vi "Particle_Setting_UI.vi"(4 "ForCalCalculaton In":T1, 6 "Analysis_Setting IN":T2 {"Analysis_Type" items=["None", "PatternMatch", "Edge Detection", "Barcode 1D", "Barcode 2D", "Clamp", "Clamp MAX", "Particle", "Histogram", "Straight Edge", "Circle", "Shape Detect", "OCR", "Contour", "ColorMatch"]}, 8 "error in (no error)":errorcluster, 9 "ProjectName":string, 10 "ROI List IN":refnum<vi>, 11 "Vision_Image":T1(plugin-control)) -> (0 "error out":errorcluster, 1 "Cancel?":bool, 2 "TempAnalysisResult":variant, 3 "Analysis_Setting":T2 {"Analysis_Type" items=["None", "PatternMatch", "Edge Detection", "Barcode 1D", "Barcode 2D", "Clamp", "Clamp MAX", "Particle", "Histogram", "Straight Edge", "Circle", "Shape Detect", "OCR", "Contour", "ColorMatch"]})   [LabVIEW 2015]
uses:
  Controls/Analysis_Setting.ctl
  Controls/Analysis_Type.ctl
  <vilib>/vision/Image Controls.llb/IMAQ Image.ctl
  Controls/_UI Command Cluster/Particle_UI Command Cluster.ctl
  Controls/Particle/Analysis_Particle_Parameter.ctl
  <vilib>/vision/NI_Vision_Development_Module.lvlib
panel:
  in  "Selected Particle":i32=2 min=-1 max=34
  in  "Simulation":bool
  out "Numeric":i32
  in  "Done":bool
  in  "Particle_UI Command":T4(ring)
  in  "Cancel":bool
  in  "ParticleTab":T5(tab)
  in  "MaxParticle":i32=1
  in  "Connectivity 4/8 (8)":bool=TRUE
  out "Selected Particle Report":T6(array[cluster]) {"Orientation" format="%.2f"; "Center of Mass"."Y" format="%.2f"; "Center of Mass"."X" format="%.2f"}
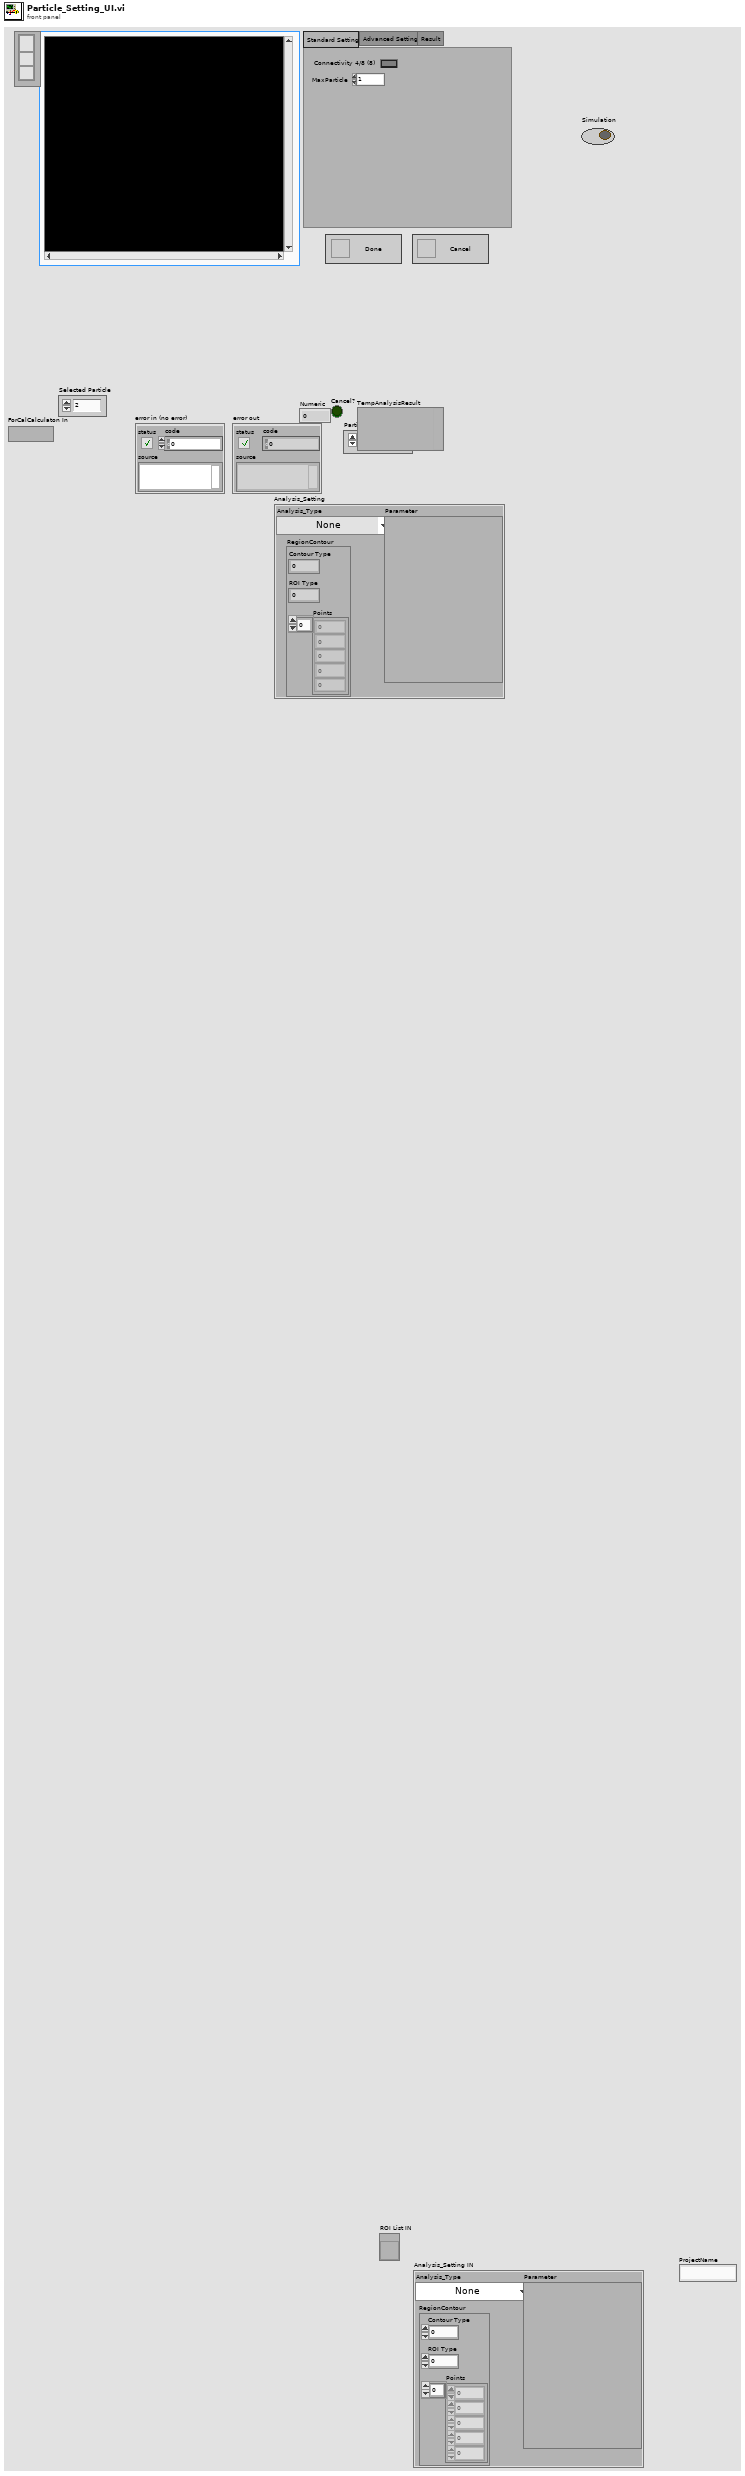
[diagram p1: front panel]
types:
  T1 = typedef "IMAQ Image.ctl" = refnum<image>
  T2 = typedef "Analysis_Setting.ctl" = cluster{"Analysis_Type":T3, "RegionContour":cluster{"Contour Type":u32, "ROI Type":u32, "Points":i32[]}, "Parameter":variant}
  T3 = typedef "Analysis_Type.ctl" = u16
  T4 = enum16{"Initialize", "Done", "Run Algorithm", "Cancel"}
  T5 = enum32{"Standard Setting", "Advanced Setting", "Result"}
  T6 = cluster{"Area":dbl, "Number of Holes":dbl, "Bounding Rect":cluster{"Left":dbl, "Top":dbl, "Right":dbl, "Bottom":dbl}, "Center of Mass":cluster{"X":dbl, "Y":dbl}, "Orientation":dbl, "Dimensions":cluster{"Width":dbl, "Height":dbl}}[]
  T7 = typedef "Particle_UI Command Cluster.ctl" = cluster{"Particle_UI Command":enum16{"Initialize", "Done", "Run Algorithm", "Cancel"}, "Selected Particle":i32, "Snap Simulation Mouse Down":bool, "Connectivity 4/8 (8)":bool, "MaxParticle":i32}
  T8 = typedef "IMAQ Line" = cluster{"Start X":i32, "Start Y":i32, "End X":i32, "End Y":i32}
  T9 = cluster{"Contour Type":u32, "ROI Type":u32, "Points":i32[]}
  T10 = typedef "Image Type" = u32
  T11 = typedef "Analysis_Particle_Parameter.ctl" = cluster{"Selected Particle":i32, "Connectivity 4/8 (8)":bool, "MaxParticle":i32}
  T12 = typedef "ROI Descriptor" = cluster{"Global Rectangle":i32[], "Contours":cluster{"ID":enum32{"External", "Internal"}, "Type":u32, "Coordinates":i32[]}[]}
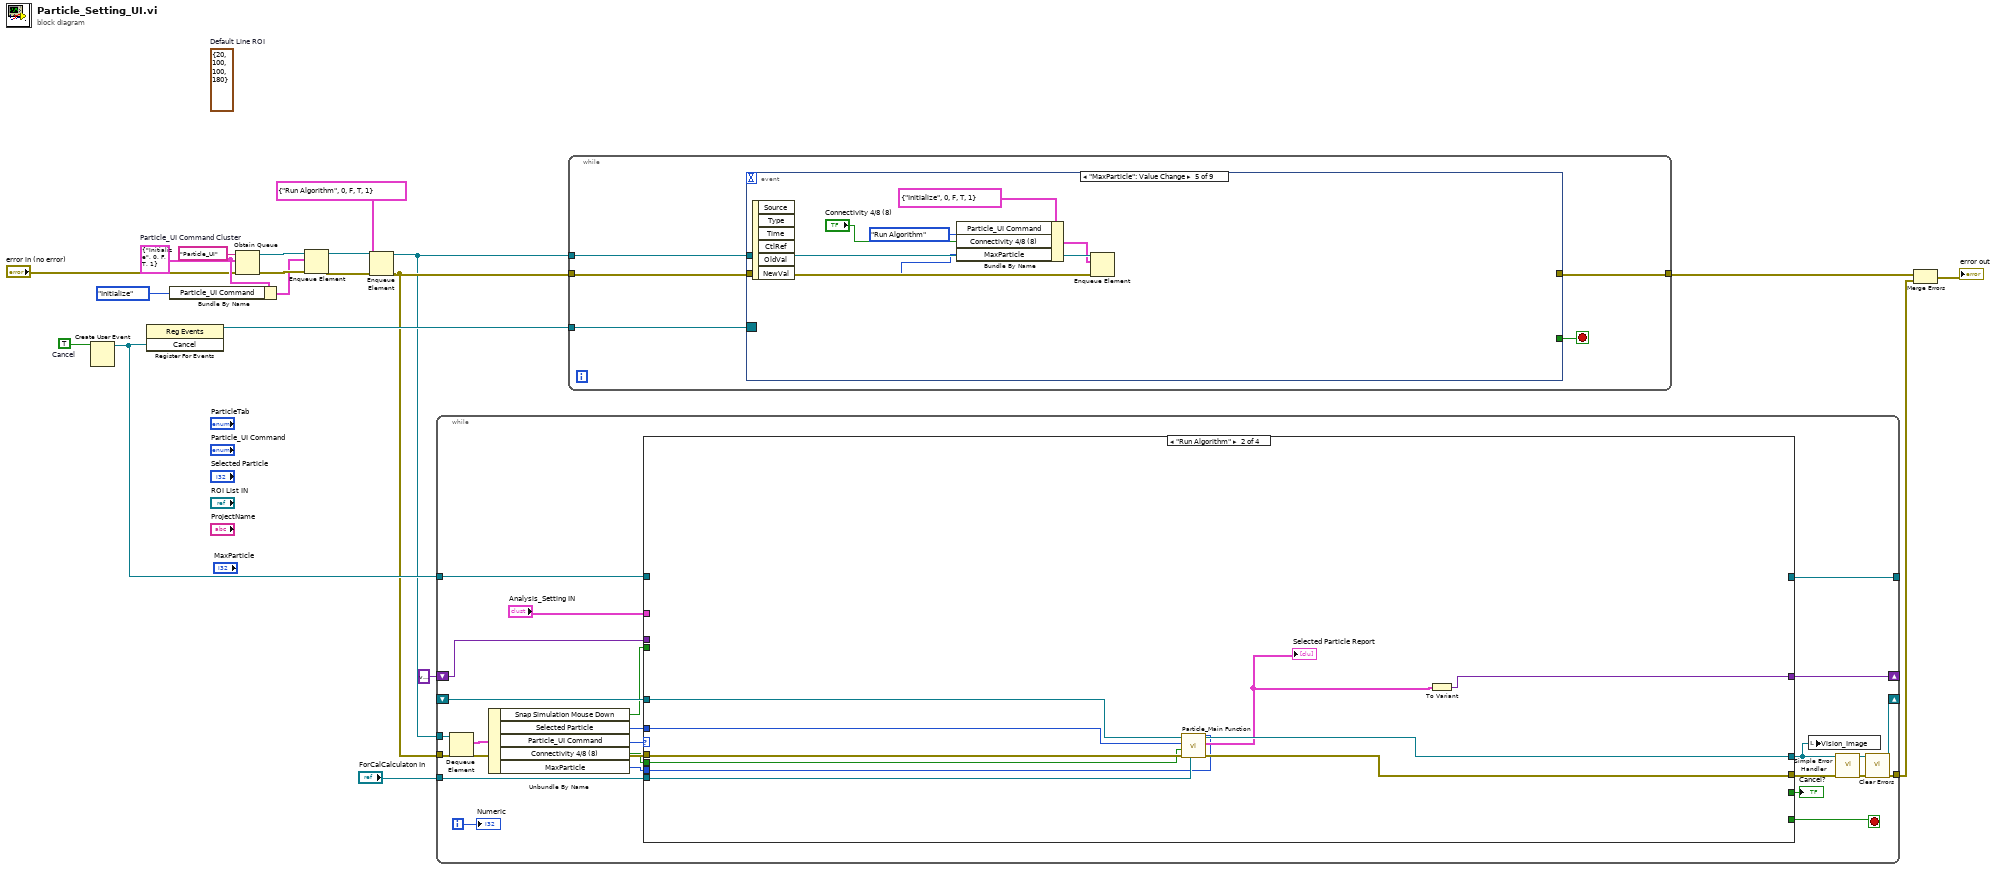
[diagram p0: block diagram]
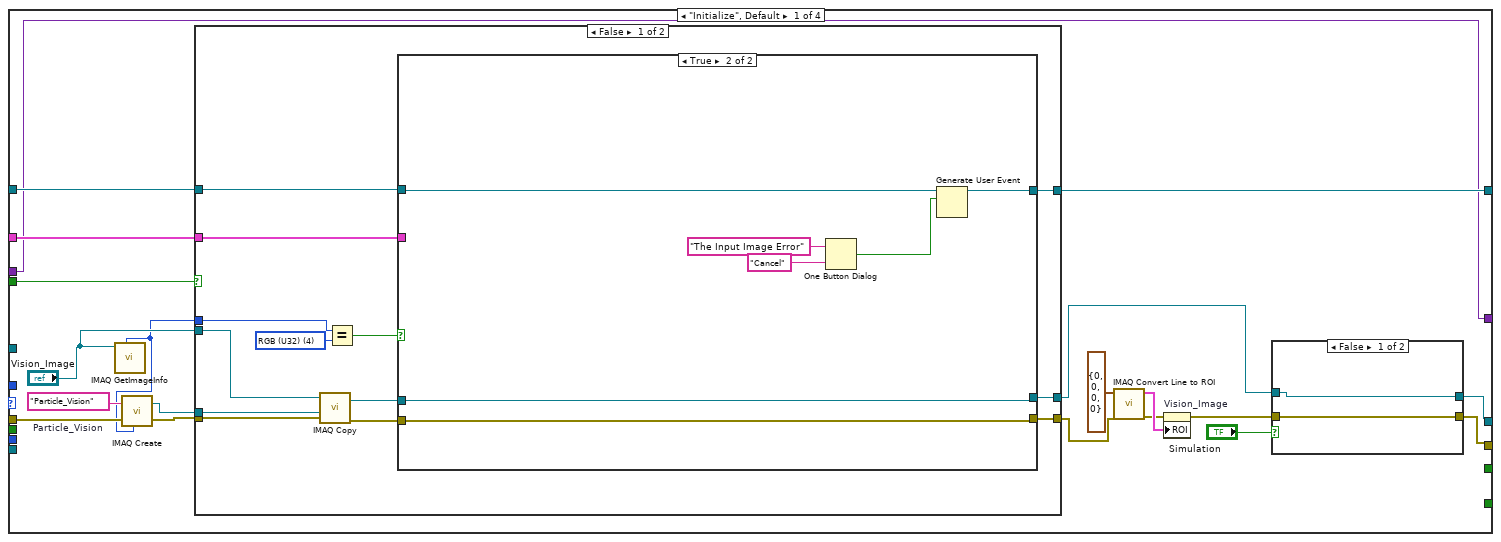
[diagram p2: hidden frame]
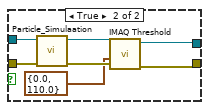
[diagram p3: hidden frame]
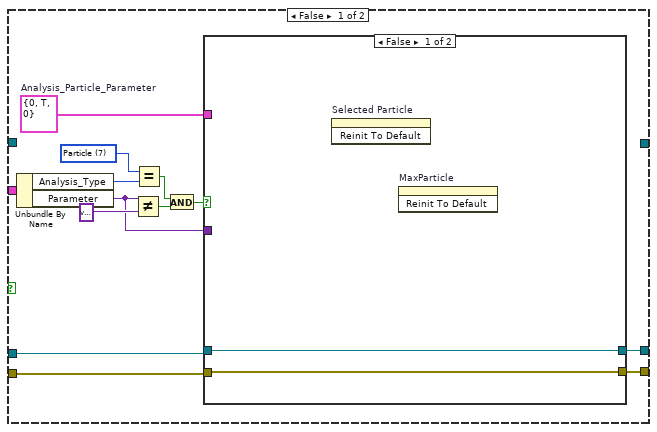
[diagram p4: hidden frame]
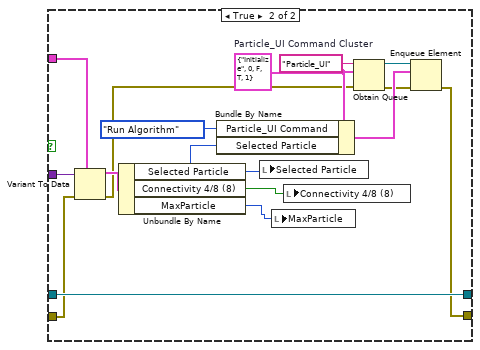
[diagram p5: hidden frame]
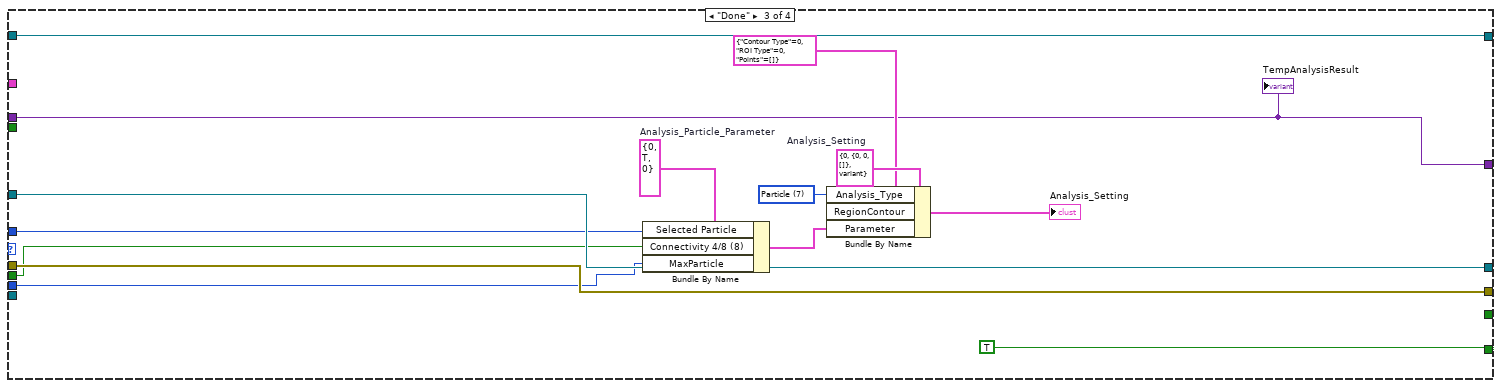
[diagram p7: hidden frame]
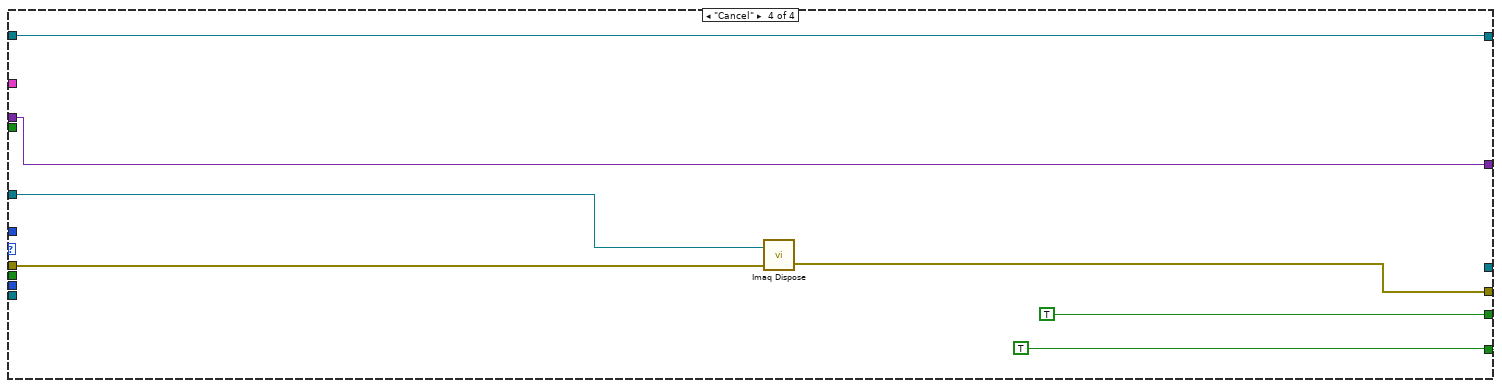
[diagram p8: hidden frame]
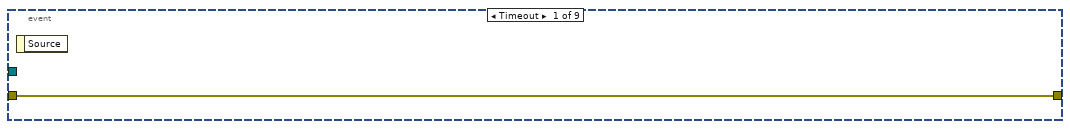
[diagram p9: hidden frame]
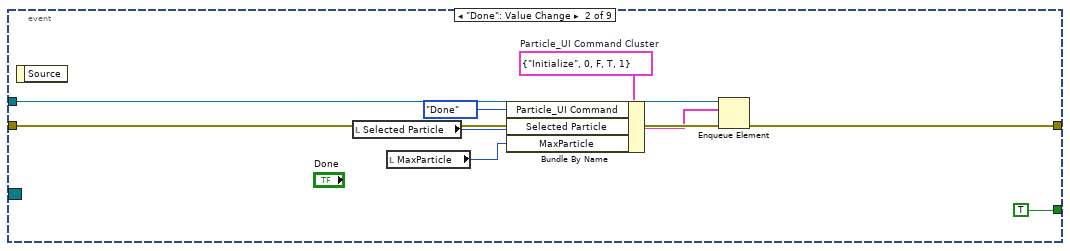
[diagram p10: hidden frame]
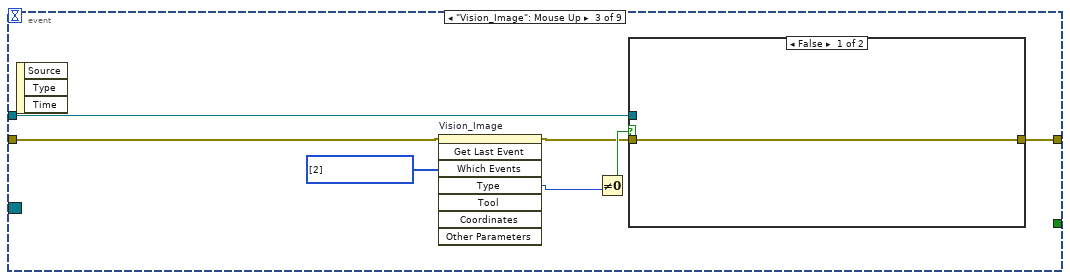
[diagram p11: hidden frame]
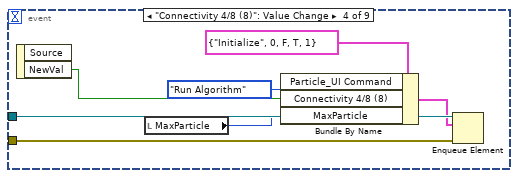
[diagram p13: hidden frame]
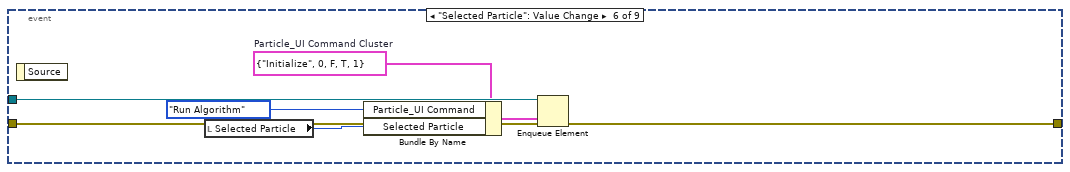
[diagram p14: hidden frame]
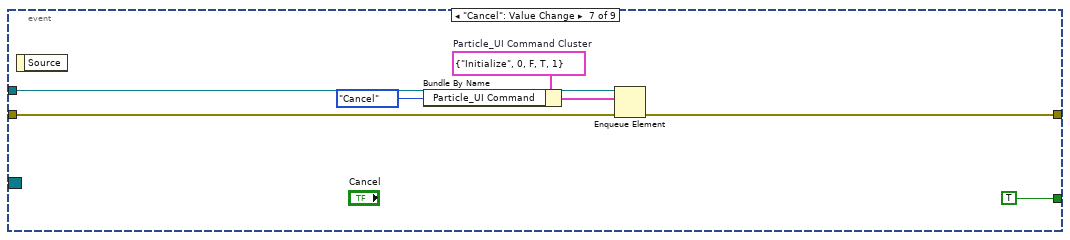
[diagram p15: hidden frame]
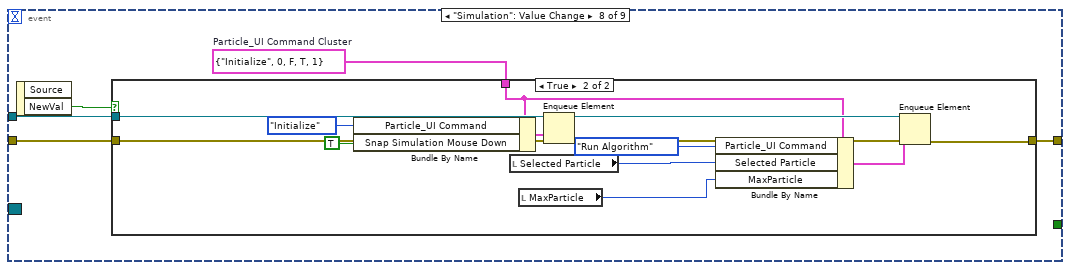
[diagram p16: hidden frame]
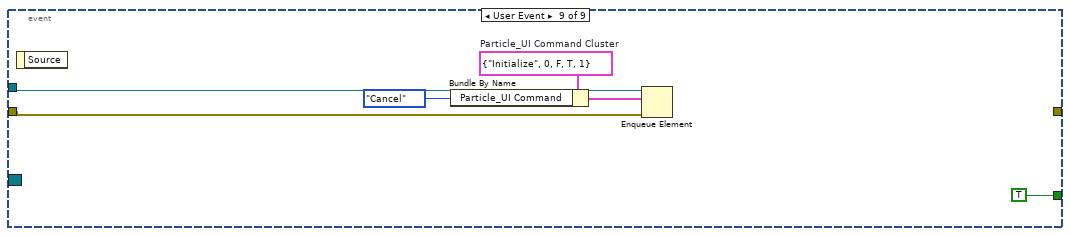
[diagram p18: hidden frame]
diagram:
  w10 = TRUE  # Cancel
  w13 = T7 {"Particle_UI Command"=enum."Initialize", "Selected Particle"=0, "Snap Simulation Mouse Down"=FALSE, "Connectivity 4/8 (8)"=TRUE, "MaxParticle"=1}  # Particle_UI Command Cluster
  (unwired) T8 {"Start X"=20, "Start Y"=100, "End X"=100, "End Y"=180}  # Default Line ROI
  n1 = Create User Event(user event datatype=w10) -> (user event=w8:refnum<user-event>)  [unwired: 1 in, 1 out]
  n2 = register-events(w8) -> (reference out=w9:refnum<event-registration>)  [unwired: 2 in, 1 out]
  n3 = Bundle By Name(cluster=w13, "Particle_UI Command"=T4."Initialize" ("Barcode 1D_UI Command")) -> (w14:T7)
  n4 = Obtain Queue(name (unnamed)="Particle_UI", element data type=w13, error in (no error)="error in (no error)") -> (queue out=w20:refnum<queue>, error out=w19:errorcluster)  [unwired: 2 in, 1 out]
  n5 = Enqueue Element(queue=w20, element=w14, error in (no error)=w19) -> (queue out=w5:refnum<queue>, error out=w7:errorcluster)  [unwired: 1 in, 1 out]
  n6 = Enqueue Element(queue=w5, element=T7 {"Particle_UI Command"=enum."Run Algorithm", "Selected Particle"=0, "Snap Simulation Mouse Down"=FALSE, "Connectivity 4/8 (8)"=TRUE, "MaxParticle"=1}, error in (no error)=w7) -> (queue out=w4:refnum<queue>, error out=w6:errorcluster)  [unwired: 1 in, 1 out]
  n7 = while {
    tunnel: w4 -> [w43]
    tunnel: w6 -> [w42]
    shift-right: [w35] -> _
    shift-left: _ -> [w37]
    tunnel: [w21] -> w16
    tunnel: w8 -> [w28]
    tunnel: [w27] -> _
    shift-right: [w26] -> _
    shift-left: variant ("Variant") -> [w25]
    tunnel: "ForCalCalculaton In" -> [w23]
    i -> [w36]
    stop <- w38 stop-if-true
    n8 = Dequeue Element(queue=w43, error in (no error)=w42) -> (element=w39:T7, error out=w40:errorcluster)  [unwired: 1 in, 2 out]
    n9 = Unbundle By Name(w39) -> ("Snap Simulation Mouse Down"=w31:bool, "Selected Particle"=w33:i32, "Particle_UI Command"=w41:T4, "Connectivity 4/8 (8)"=w24:bool, "MaxParticle"=w22:i32)
    n10 = case shown="\"Run Algorithm\"" w41 {
      tunnel: w40 -> [w62 w135 w147 w154]
      tunnel: [w49 w131 w147 w153] -> w30
      tunnel: [_ _ TRUE TRUE] -> w38
      tunnel: [w50 w132 w148 _] -> w35
      tunnel: w37 -> [_ w133 w148 w155]
      tunnel: [_ _ _ TRUE] -> w34
      tunnel: w33 -> [_ w134 w141 _]
      tunnel: "Analysis_Setting IN" -> [w61 _ _ _]
      tunnel: w31 -> [w53 _ _ _]
      tunnel: w28 -> [w48 _ w139 w151]
      tunnel: [w47 _ w139 w151] -> w27
      tunnel: [w44 w129 w138 w150] -> w26
      tunnel: w25 -> [w44 _ w138 w150]
      tunnel: w24 -> [_ w128 w137 _]
      tunnel: w23 -> [_ w127 _ _]
      tunnel: w22 -> [_ w126 w136 _]
      frame "Initialize", Default {
        w63 = "Particle_Vision"  # Particle_Vision
        n11 = call "IMAQ GetImageInfo"("Image"="Vision_Image") -> ("Image Type"=w45:T10)  [unwired: 3 in, 7 out]
        n12 = call "IMAQ Create"("Image Name"=w63, "Image Type"=w45, "error in (no error)"=w62) -> ("New Image"=w51:T1, "error out"=w52:errorcluster)  [unwired: 2 in]
        n13 = case shown="False" w53 {
          tunnel: w61 -> [w85 _]
          tunnel: [w84 w125] -> w54
          tunnel: [w83 w124] -> w55
          tunnel: w52 -> [w82 w124]
          tunnel: w51 -> [w81 w125]
          tunnel: w48 -> [w76 _]
          tunnel: [w75 _] -> w47
          tunnel: "Vision_Image" -> [w74 _]
          tunnel: w45 -> [w73 _]
          frame False {
            w78 = T10 4 items=["Grayscale (U8)", "Grayscale (I16)", "Grayscale (SGL)", "Complex (CSG)", "RGB (U32)", "HSL (U32)", "RGB (U64)", "Grayscale (U16)"] ("y")
            n14 = call "IMAQ Copy"("error in (no error)"=w82, "Image Dst"=w81, "Image Src"=w74) -> ("error out"=w80:errorcluster, "Image Dst Out"=w79:T1)  [unwired: 3 in]
            n15 = Equal?(x=w73, y=w78) -> (x = y?=w77:bool)
            n16 = case shown="True" w77 {
              tunnel: w85 -> [w91 _]
              tunnel: [w89 w117] -> w84
              tunnel: [w88 w118] -> w83
              tunnel: w80 -> [w87 w118]
              tunnel: w79 -> [w86 w117]
              tunnel: w76 -> [_ w120]
              tunnel: [_ w119] -> w75
              frame False {
                w90 = T11 {"Selected Particle"=0, "Connectivity 4/8 (8)"=TRUE, "MaxParticle"=0}  # Analysis_Particle_Parameter
                w96 = T3 7 items=["None", "PatternMatch", "Edge Detection", "Barcode 1D", "Barcode 2D", "Clamp", "Clamp MAX", "Particle", "Histogram", "Straight Edge", "Circle", "Shape Detect", "OCR", "Contour", "ColorMatch"] ("x")
                n17 = Unbundle By Name(w91) -> ("Analysis_Type"=w95:T3, "Parameter"=w92:variant)
                n18 = Not Equal?(x=w92, y=variant) -> (x != y?=w97:bool)
                n19 = Equal?(x=w96, y=w95) -> (x = y?=w98:bool)
                n20 = And(x=w98, y=w97) -> (x .and. y?=w93:bool)
                n21 = case shown="False" w93 {
                  tunnel: w87 -> [w99 w105]
                  tunnel: w86 -> [w100 w106]
                  tunnel: [w100 w106] -> w89
                  tunnel: [w99 w103] -> w88
                  tunnel: w92 -> [_ w116]
                  tunnel: w90 -> [_ w114]
                  frame False {
                    n22 = invoke on="Selected Particle" class="DigNum (strict)" method="Reinit To Default"() -> ()  [unwired: 3 in, 3 out]
                    n23 = invoke on="MaxParticle" class="DigNum (strict)" method="Reinit To Default"() -> ()  [unwired: 3 in, 3 out]
                  }
                  frame True {
                    w113 = T7 {"Particle_UI Command"=enum."Initialize", "Selected Particle"=0, "Snap Simulation Mouse Down"=FALSE, "Connectivity 4/8 (8)"=TRUE, "MaxParticle"=1}  # Particle_UI Command Cluster
                    n24 = Variant To Data(error in=w105, type=w114, Variant=w116) -> (data=w115:T11, error out=w104:errorcluster)
                    n25 = Unbundle By Name(w115) -> ("Selected Particle"=w107:i32, "Connectivity 4/8 (8)"=w102:bool, "MaxParticle"=w101:i32)
                    n26 = Bundle By Name(cluster=w113, "Particle_UI Command"=T4."Run Algorithm" ("Barcode 1D_UI Command"), "Selected Particle"=w107) -> (w112:T7)
                    n27 = local write "Selected Particle"(w107) -> ()
                    n28 = local write "MaxParticle"(w101) -> ()
                    n29 = local write "Connectivity 4/8 (8)"(w102) -> ()
                    n30 = Obtain Queue(name (unnamed)="Particle_UI", element data type=w113, error in (no error)=w104) -> (queue out=w108:refnum<queue>, error out=w109:errorcluster)  [unwired: 2 in, 1 out]
                    n31 = Enqueue Element(queue=w108, element=w112, error in (no error)=w109) -> (error out=w103:errorcluster)  [unwired: 1 in, 2 out]
                  }
                }
              }
              frame True {
                n32 = One Button Dialog(message="The Input Image Error", button name ("OK")="Cancel") -> (true=w121:bool)
                n33 = Generate User Event(user event=w120, event data cluster=w121) -> (user event out=w119:refnum<user-event>)  [unwired: 2 in, 1 out]
              }
            }
          }
          frame True {
          }
        }
        n34 = call "IMAQ Convert Line to ROI"("error in (no error)"=w55, "Line"=T8 {"Start X"=0, "Start Y"=0, "End X"=0, "End Y"=0}) -> ("error out"=w56:errorcluster, "ROI Descriptor"=w57:T12)  [unwired: 7 in]
        n35 = property on="Vision_Image" class="ImageControl"(error in=w56, "ROI"=w57) -> (error out=w59:errorcluster)  [unwired: 1 in, 1 out]
        n36 = case shown="False" "Simulation" {
          tunnel: [w65 w67] -> w49
          tunnel: [w64 w68] -> w50
          tunnel: w59 -> [w65 w72]
          tunnel: w54 -> [w64 w71]
          frame False {
          }
          frame True {
            n37 = call "Particle_Simulaation.vi"("error in (no error)"=w72, "Refnum in"=w71) -> ("error out"=w69:errorcluster, "Refnum out"=w70:T1)  [unwired: 8 in]
            n38 = call "IMAQ Threshold"("error in (no error)"=w69, "Range"=cluster{"Lower value":sgl, "Upper value":sgl} {"Lower value"=0.0, "Upper value"=110.0}, "Image Src"=w70) -> ("error out"=w67:errorcluster, "Image Dst Out"=w68:T1)  [unwired: 7 in]
          }
        }
      }
      frame "Run Algorithm" {
        n39 = call "Particle_Main Function.vi"("ForCalCalculaton In"=w127, "MAXParticle"=w126, "error in (no error)"=w135, "Connectivity 4/8 (8)"=w128, "Selected Particle"=w134, "Refnum in"=w133) -> ("error out"=w131:errorcluster, "Particle Report"=w130:T6, "Refnum out"=w132:T1)  [unwired: 1 in, 2 out]
        "Selected Particle Report" <- w130
        n40 = To Variant(anything=w130) -> (Variant=w129:variant)
      }
      frame "Done" {
        w143 = T11 {"Selected Particle"=0, "Connectivity 4/8 (8)"=TRUE, "MaxParticle"=0}  # Analysis_Particle_Parameter
        w145 = T3 7 items=["None", "PatternMatch", "Edge Detection", "Barcode 1D", "Barcode 2D", "Clamp", "Clamp MAX", "Particle", "Histogram", "Straight Edge", "Circle", "Shape Detect", "OCR", "Contour", "ColorMatch"] ("Analysis_Type")
        w146 = T2 {"Analysis_Type"=0, "RegionContour"={"Contour Type"=0, "ROI Type"=0, "Points"=[]}, "Parameter"=variant}  # Analysis_Setting
        n41 = Bundle By Name(cluster=w143, "Selected Particle"=w141, "Connectivity 4/8 (8)"=w137, "MaxParticle"=w136) -> (w142:T11)
        n42 = Bundle By Name(cluster=w146, "Analysis_Type"=w145, "RegionContour"=T9 {"Contour Type"=0, "ROI Type"=0, "Points"=[]}, "Parameter"=w142) -> (→"Analysis_Setting":T2)
        "TempAnalysisResult" <- w138
      }
      frame "Cancel" {
        n43 = call "Imaq Dispose"("Image"=w155, "error in (no error)"=w154) -> ("error out"=w153:errorcluster)  [unwired: 4 in]
      }
    }
    "Cancel?" <- w34
    n44 = local write "Vision_Image"(w35) -> ()
    n45 = call <vilib>:"Simple Error Handler.vi"("error in (no error)"=w30) -> ("error out"=w29:errorcluster)  [unwired: 4 in, 4 out]
    n46 = call <vilib>:"Clear Errors.vi"("error in (no error)"=w29) -> ("error out"=w21:errorcluster)  [unwired: 5 in, 1 out]
    "Numeric" <- w36
  }
  n47 = while {
    tunnel: w4 -> [w161]
    tunnel: w6 -> [w160]
    tunnel: [w158] -> w17
    tunnel: w9 -> [w157]
    stop <- w159 stop-if-true
    n48 = event shown="[4] \"MaxParticle\": Value Change" {
      selector: w157 -> [_ _ _ _ _ _ _ _ _]
      dyn-events: _ -> [_ _ _ _ _ _ _ _ _]
      timeout: _ -> [_ _ _ _ _ _ _ _ _]
      tunnel: w161 -> [_ w171 w178 w187 w194 w201 w208 w213 w229]
      tunnel: w160 -> [w162 w170 w175 w186 w193 w200 w207 w212 w228]
      tunnel: [_ TRUE _ _ _ _ TRUE _ TRUE] -> w159
      tunnel: [w162 w169 w172 _ _ w199 w205 w210 _] -> w158
      event Timeout {
        n49 = event-data() -> ()  [unwired: 1 in, 1 out]
      }
      event "Done": Value Change {
        w168 = T7 {"Particle_UI Command"=enum."Initialize", "Selected Particle"=0, "Snap Simulation Mouse Down"=FALSE, "Connectivity 4/8 (8)"=TRUE, "MaxParticle"=1}  # Particle_UI Command Cluster
        n50 = event-data() -> ()  [unwired: 1 in, 1 out]
        n51 = local read "Selected Particle"() -> (w164:i32)
        n52 = local read "MaxParticle"() -> (w163:i32)
        n53 = Bundle By Name(cluster=w168, "Particle_UI Command"=T4."Done" ("Edge Detection_UI Command"), "Selected Particle"=w164, "MaxParticle"=w163) -> (w166:T7)
        n54 = Enqueue Element(queue=w171, element=w166, error in (no error)=w170) -> (error out=w169:errorcluster)  [unwired: 1 in, 2 out]
      }
      event "Vision_Image": Mouse Up {
        w176 = i32[] [2] items=["No Event"=0, "Click Event"=1, "Draw Event"=2, "Size Event"=4, "Scroll Event"=5, "Double Click Event"=8] ("Which Events")
        n55 = event-data() -> ()  [unwired: 1 in, 3 out]
        n56 = invoke on="Vision_Image" class="ImageControl" method="Get Last Event"(error in=w175, "Which Events"=w176) -> (error out=w174:errorcluster, "Type"=w173:i32)  [unwired: 6 in, 6 out]
        n57 = Not Equal To 0?(x=w173) -> (x != 0?=w177:bool)
        n58 = case shown="False" w177 {
          tunnel: w178 -> [_ _]
          tunnel: w174 -> [w179 w180]
          tunnel: [w179 w180] -> w172
          frame False {
          }
          frame True {
          }
        }
      }
      event "Connectivity 4/8 (8)": Value Change {
        n59 = event-data() -> ("NewVal"=w182:bool)  [unwired: 1 in, 1 out]
        n60 = local read "MaxParticle"() -> (w181:i32)
        n61 = Bundle By Name(cluster=T7 {"Particle_UI Command"=enum."Initialize", "Selected Particle"=0, "Snap Simulation Mouse Down"=FALSE, "Connectivity 4/8 (8)"=TRUE, "MaxParticle"=1} ("element"), "Particle_UI Command"=T4."Run Algorithm", "Connectivity 4/8 (8)"=w182, "MaxParticle"=w181) -> (w184:T7)
        n62 = Enqueue Element(queue=w187, element=w184, error in (no error)=w186) -> ()  [unwired: 1 in, 3 out]
      }
      event "MaxParticle": Value Change {
        n63 = event-data() -> ("NewVal"=w189:i32)  [unwired: 1 in, 5 out]
        n64 = Bundle By Name(cluster=T7 {"Particle_UI Command"=enum."Initialize", "Selected Particle"=0, "Snap Simulation Mouse Down"=FALSE, "Connectivity 4/8 (8)"=TRUE, "MaxParticle"=1} ("element"), "Particle_UI Command"=T4."Run Algorithm", "Connectivity 4/8 (8)"="Connectivity 4/8 (8)", "MaxParticle"=w189) -> (w191:T7)
        n65 = Enqueue Element(queue=w194, element=w191, error in (no error)=w193) -> ()  [unwired: 1 in, 3 out]
      }
      event "Selected Particle": Value Change {
        w198 = T7 {"Particle_UI Command"=enum."Initialize", "Selected Particle"=0, "Snap Simulation Mouse Down"=FALSE, "Connectivity 4/8 (8)"=TRUE, "MaxParticle"=1}  # Particle_UI Command Cluster
        n66 = event-data() -> ()  [unwired: 1 in, 1 out]
        n67 = local read "Selected Particle"() -> (w195:i32)
        n68 = Bundle By Name(cluster=w198, "Particle_UI Command"=T4."Run Algorithm" ("Barcode 1D_UI Command"), "Selected Particle"=w195) -> (w196:T7)
        n69 = Enqueue Element(queue=w201, element=w196, error in (no error)=w200) -> (error out=w199:errorcluster)  [unwired: 1 in, 2 out]
      }
      event "Cancel": Value Change {
        w203 = T7 {"Particle_UI Command"=enum."Initialize", "Selected Particle"=0, "Snap Simulation Mouse Down"=FALSE, "Connectivity 4/8 (8)"=TRUE, "MaxParticle"=1}  # Particle_UI Command Cluster
        n70 = event-data() -> ()  [unwired: 1 in, 1 out]
        n71 = Bundle By Name(cluster=w203, "Particle_UI Command"=T4."Cancel" ("Barcode 1D_UI Command")) -> (w202:T7)
        n72 = Enqueue Element(queue=w208, element=w202, error in (no error)=w207) -> (error out=w205:errorcluster)  [unwired: 1 in, 2 out]
      }
      event "Simulation": Value Change {
        w209 = T7 {"Particle_UI Command"=enum."Initialize", "Selected Particle"=0, "Snap Simulation Mouse Down"=FALSE, "Connectivity 4/8 (8)"=TRUE, "MaxParticle"=1}  # Particle_UI Command Cluster
        n73 = event-data() -> ("NewVal"=w211:bool)  [unwired: 1 in, 1 out]
        n74 = case shown="True" w211 {
          tunnel: w213 -> [_ w227]
          tunnel: w212 -> [w214 w226]
          tunnel: w209 -> [_ w220]
          tunnel: [w214 w221] -> w210
          frame False {
          }
          frame True {
            n75 = Bundle By Name(cluster=w220, "Particle_UI Command"=T4."Initialize" ("Barcode 1D_UI Command"), "Snap Simulation Mouse Down"=TRUE) -> (w224:T7)
            n76 = local read "Selected Particle"() -> (w217:i32)
            n77 = local read "MaxParticle"() -> (w215:i32)
            n78 = Enqueue Element(queue=w227, element=w224, error in (no error)=w226) -> (queue out=w223:refnum<queue>, error out=w222:errorcluster)  [unwired: 1 in, 1 out]
            n79 = Bundle By Name(cluster=w220, "Particle_UI Command"=T4."Run Algorithm", "Selected Particle"=w217, "MaxParticle"=w215) -> (w219:T7)
            n80 = Enqueue Element(queue=w223, element=w219, error in (no error)=w222) -> (error out=w221:errorcluster)  [unwired: 1 in, 2 out]
          }
        }
      }
      event User Event {
        w231 = T7 {"Particle_UI Command"=enum."Initialize", "Selected Particle"=0, "Snap Simulation Mouse Down"=FALSE, "Connectivity 4/8 (8)"=TRUE, "MaxParticle"=1}  # Particle_UI Command Cluster
        n81 = event-data() -> ()  [unwired: 1 in, 1 out]
        n82 = Bundle By Name(cluster=w231, "Particle_UI Command"=T4."Cancel" ("Barcode 1D_UI Command")) -> (w230:T7)
        n83 = Enqueue Element(queue=w229, element=w230, error in (no error)=w228) -> ()  [unwired: 1 in, 3 out]
      }
    }
  }
  n84 = Merge Errors(w17, w16) -> (→"error out":errorcluster)
